vi "CreatePath_WriteGlobal_Example.vi"   [LabVIEW 2019]
uses:
  SubVI/StoreTrajectory_GlobalVariable.vi
panel:
  # "Create Trajectory and Write to Global Variable"
  # "See block diagram"
types:
  T1 = typedef "PathPlanner24.lvlib/PathPlannerTrajectory.ctl" = cluster{"States":T2[]}
  T2 = typedef "PathPlanner24.lvlib/PathPlannerTrajectoryState.ctl" = cluster{"TimeSeconds":dbl, "VelocityMPS":dbl, "AccerationMpsSq":dbl, "HeadingAngularVelRadPerSec":dbl, "PositionMeters":T3, "Heading":T4, "TargetHolonomicRotation":T4, "CurvatureRadPerMeter":dbl, "PathPlannerConstraints":T5, "DeltaPos":dbl}
  T3 = typedef "Trajectory_Library.lvlib/TRANSLATION2D.ctl" = cluster{"X":dbl, "Y":dbl}
  T4 = typedef "Trajectory_Library.lvlib/ROTATION2D.ctl" = cluster{"VALUE":dbl, "COS":dbl, "SIN":dbl}
  T5 = typedef "PathPlanner24.lvlib/PathPlannerPathConstraints.ctl" = cluster{"MaxVelocityMps;":dbl, "MaxAccelerationMpsSq;":dbl, "MaxAngularVelRadPsEc;":dbl, "MaxAngularAccRadPSecSq":dbl, "Exists":bool}
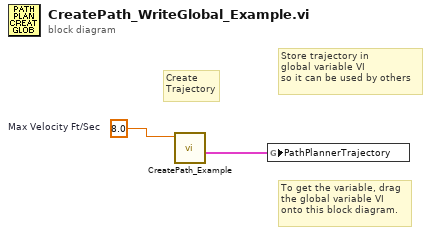
[diagram p0: block diagram]
diagram:
  w2 = 8.0  # Max Velocity Ft/Sec
  # "To get the variable, drag\nthe global variable VI\nonto this block diagram."
  # "Create\nTrajectory"
  # "Store trajectory in\nglobal variable VI\nso it can be used by others"
  n1 = call "CreatePath_Example.vi"("Max Velocity M/S"=w2) -> ("PathPlannerTrajectory"=w1:T1)  [unwired: 8 in, 2 out]
  n2 = global write "StoreTrajectory_GlobalVariable.vi" "PathPlannerTrajectory"(w1) -> ()
